vi "pruebas.vi"() -> ()   [LabVIEW 2021, in "Test_VIs.lvlib"]
uses:
  Test_VIs.lvlib
panel:
  out "Minutos":dbl
  in  "milliseconds to wait 2":u32
  in  "Entrada digital Bitron":bool
  in  "Run Program":bool
  in  "Reset temp":bool
  out "t ensayo (s) 2":u64
  out "Minutos totales":dbl
  out "Horas 2":dbl
  out "días 2":dbl
  out "segundos":dbl
  out "Medios ciclos totales":dbl
  out "concatenated string":string
  out "segundos":dbl
  out "días":dbl
  out "Horas":dbl
  out "Minutos":dbl
  out "t ensayo (s)":u64
  out "Time Stamp 2":timestamp format="%<%H:%M:%S>T"
  out "x-y":dbl
  in  "milliseconds to wait":u32=1000
  out "Time Stamp":timestamp format="%<%H:%M:%S>T"
  in  "stop":bool
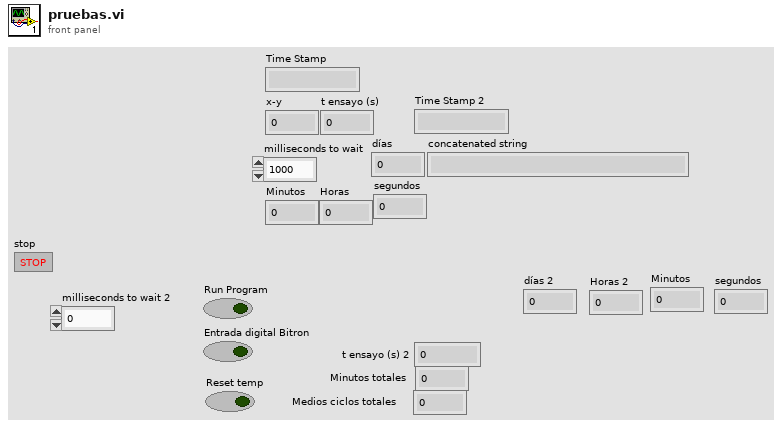
[diagram p1: front panel]
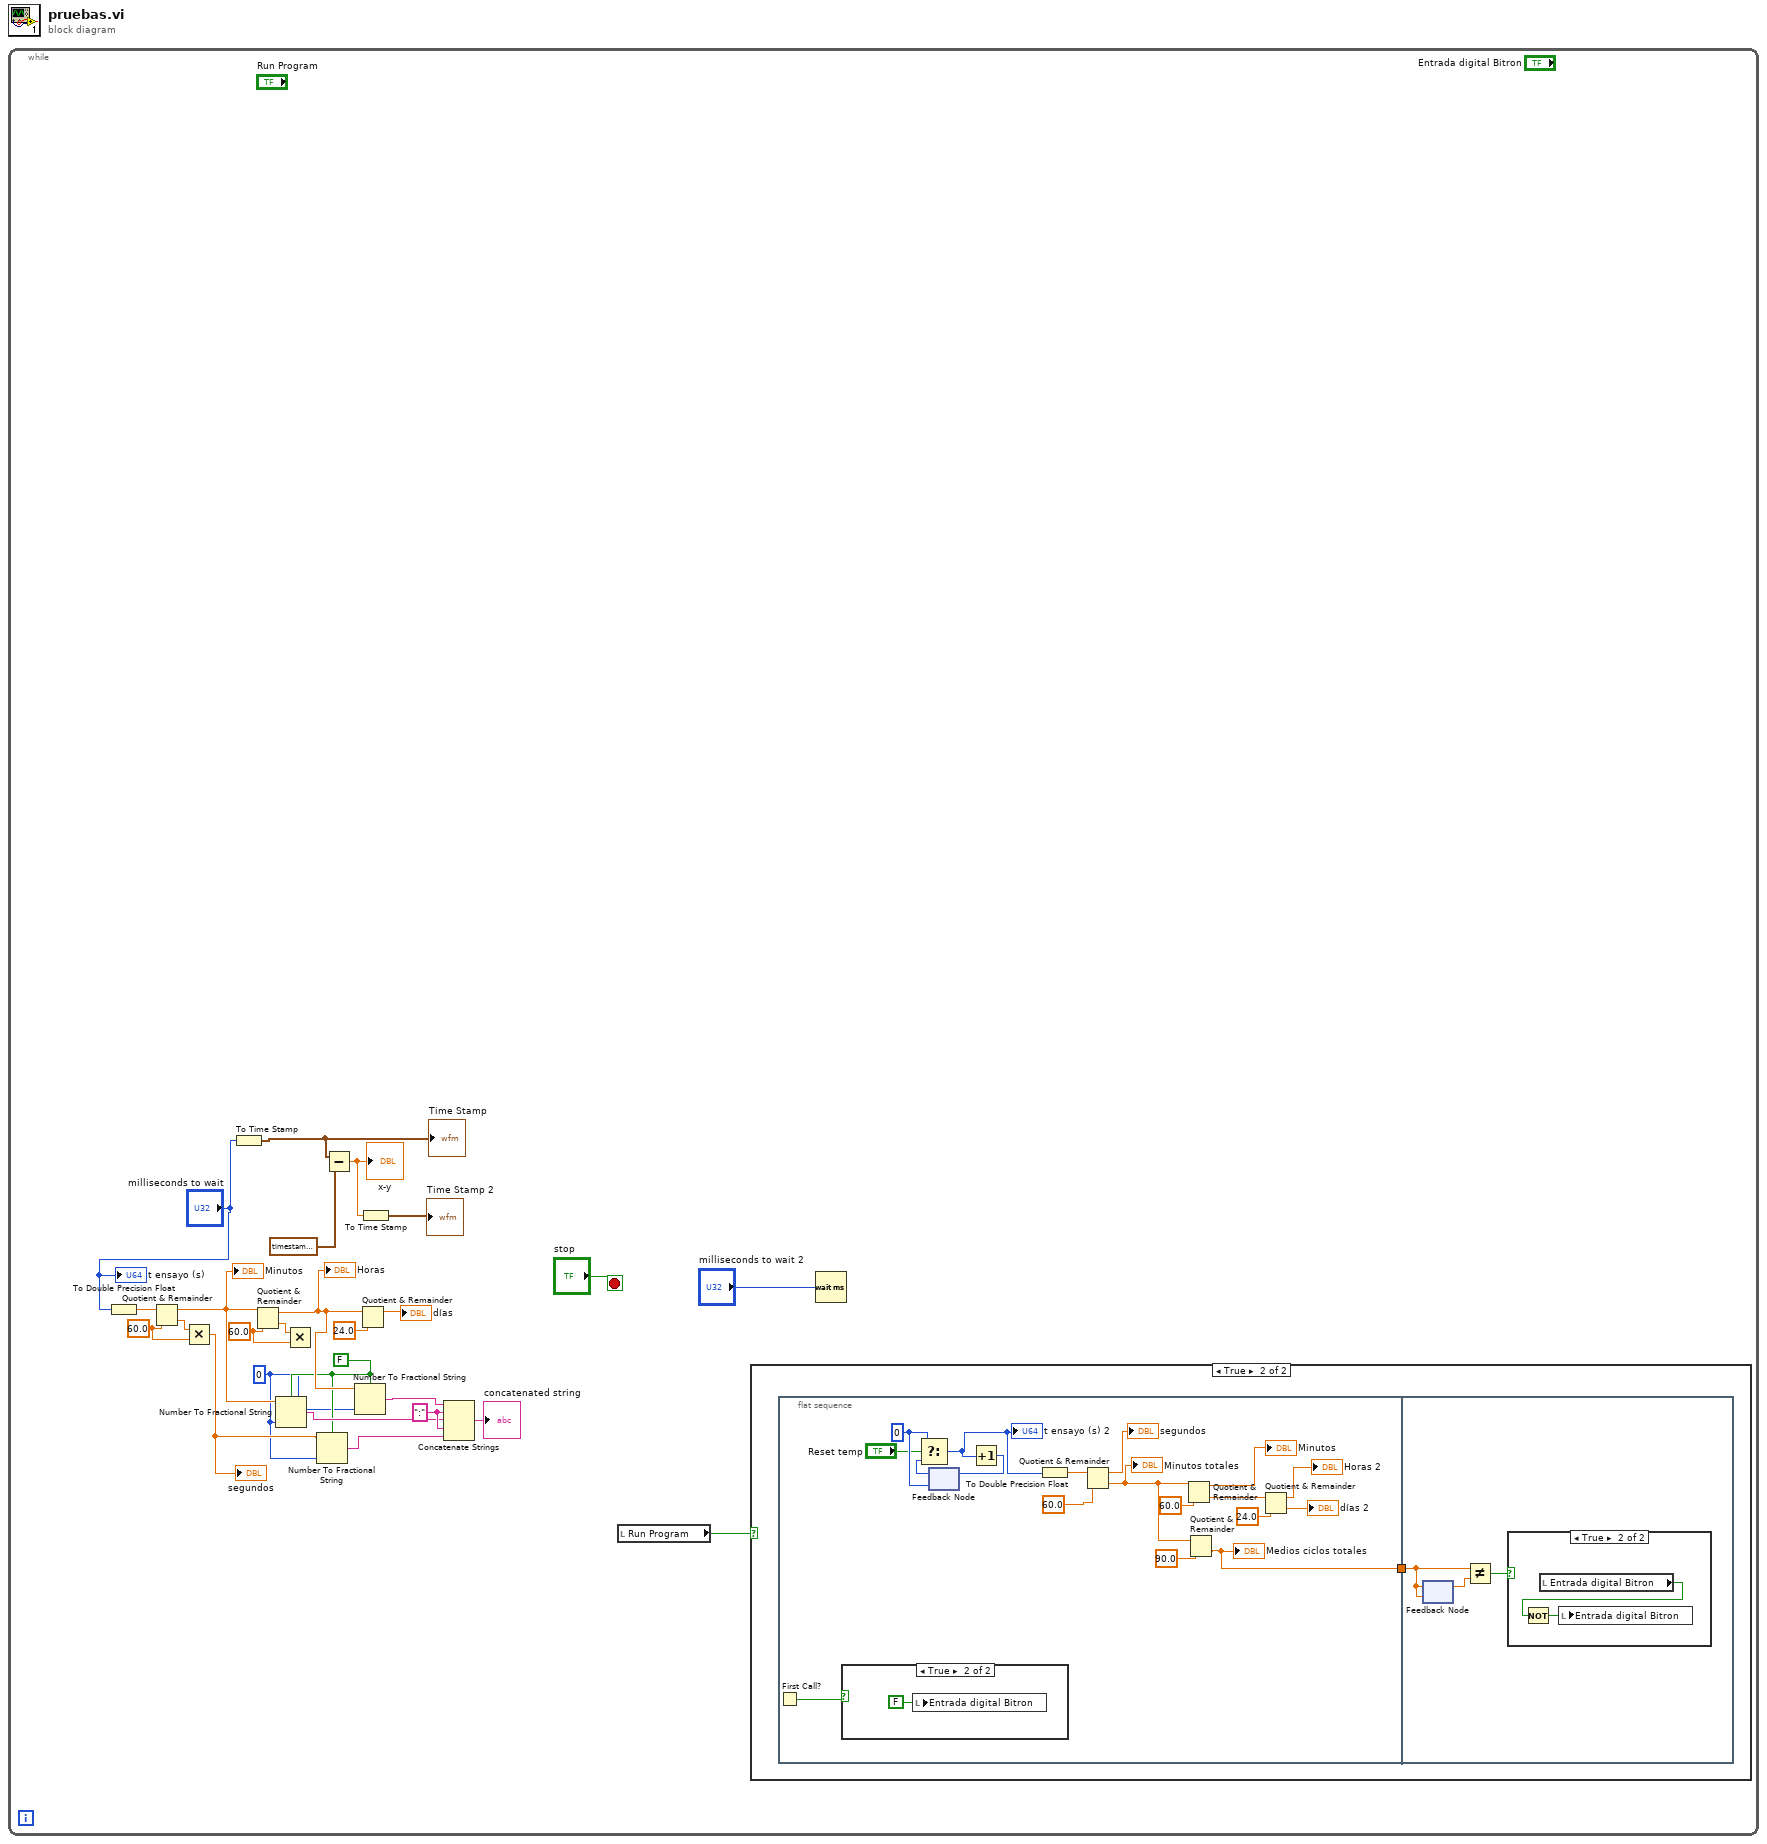
[diagram p0: block diagram]
diagram:
  n1 = while {
    stop <- "stop" stop-if-true
    w3 = i16 0 ("precision (6)")
    w4 = FALSE ("use system decimal point (T)")
    w13 = ":" ("string")
    w17 = 60.0 ("y")
    w18 = 60.0 ("y")
    n2 = To Double Precision Float(number="milliseconds to wait") -> (double precision float=w20:dbl)
    n3 = Quotient & Remainder(x=w20, y=w18) -> (x-y*floor(x/y)=w8:dbl, floor(x/y)=w19:dbl)
    "Minutos" <- w8
    n4 = Multiply(x=w19, y=w18) -> (x*y=w7:dbl)
    "segundos" <- w7
    n5 = To Time Stamp(1:"milliseconds to wait") -> (0:w24:timestamp)
    "Time Stamp" <- w24
    n6 = Quotient & Remainder(x=w8, y=w17) -> (x-y*floor(x/y)=w10:dbl, floor(x/y)=w16:dbl)
    "Horas" <- w10
    n7 = Number To Fractional String(use system decimal point (T)=w4, number=w8, precision (6)=w3) -> (F-format string=w6:string)  [unwired: 1 in]
    n8 = Multiply(x=w16, y=w17) -> ()  [unwired: 1 out]
    n9 = Number To Fractional String(use system decimal point (T)=w4, number=w7, precision (6)=w3) -> (F-format string=w5:string)  [unwired: 1 in]
    n10 = Subtract(x=w24, y=timestamp(79200 s since 1904-01-01)) -> (x-y=w22:dbl)
    "x-y" <- w22
    n11 = Number To Fractional String(use system decimal point (T)=w4, number=w10, precision (6)=w3) -> (F-format string=w9:string)  [unwired: 1 in]
    n12 = Quotient & Remainder(x=w10, y=24.0) -> (x-y*floor(x/y)=→"días":dbl)  [unwired: 1 out]
    n13 = To Time Stamp(1:w22) -> (0:→"Time Stamp 2":timestamp)
    n14 = Concatenate Strings(w9, w13, w6, w13, w5) -> (→"concatenated string":string)
    n15 = local read "Run Program"() -> (w2:bool)
    n16 = case shown="True" w2 {
      frame False {
      }
      frame True {
        n17 = flat-sequence {
          tunnel: [w29] -> w26
          tunnel: w26 -> [w48]
          frame #0 {
            w37 = u64 0 ("t")
            n18 = First Call?() -> (First Call?: T/F=w44:bool)
            n19 = case shown="True" w44 {
              frame False {
              }
              frame True {
                n20 = local write "Entrada digital Bitron"(FALSE ("Entrada digital Bitron")) -> ()
              }
            }
            n21 = feedback #1(w37) -> (w35:u64)
            n22 = Select(t=w37, s="Reset temp", f=w35) -> (s? t:f=w38:u64)
            "t ensayo (s) 2" <- w38
            n23 = Increment(x=w38) -> (x+1=w36:u64)
            n24 = feedback-in #1(w36) -> ()
            n25 = To Double Precision Float(number=w38) -> (double precision float=w39:dbl)
            n26 = Quotient & Remainder(x=w39, y=60.0) -> (x-y*floor(x/y)=→"segundos":dbl, floor(x/y)=w33:dbl)
            "Minutos totales" <- w33
            n27 = Quotient & Remainder(x=w33, y=60.0) -> (x-y*floor(x/y)=→"Minutos":dbl, floor(x/y)=w32:dbl)
            n28 = Quotient & Remainder(x=w33, y=90.0) -> (floor(x/y)=w29:dbl)  [unwired: 1 out]
            "Medios ciclos totales" <- w29
            n29 = Quotient & Remainder(x=w32, y=24.0) -> (x-y*floor(x/y)=→"Horas 2":dbl, floor(x/y)=→"días 2":dbl)
          }
          frame #1 {
            n30 = feedback-in #2(w48) -> ()
            n31 = feedback #2(w48) -> (w47:dbl)
            n32 = Not Equal?(x=w48, y=w47) -> (x != y?=w46:bool)
            n33 = case shown="True" w46 {
              frame False {
              }
              frame True {
                n34 = local read "Entrada digital Bitron"() -> (w49:bool)
                n35 = Not(x=w49) -> (.not. x?=w50:bool)
                n36 = local write "Entrada digital Bitron"(w50) -> ()
              }
            }
          }
        }
      }
    }
    n37 = Wait (ms)(milliseconds to wait="milliseconds to wait 2") -> ()  [unwired: 1 out]
    "t ensayo (s)" <- "milliseconds to wait"
  }
